vi "TiePie.Scp.ScpIsRunning.vi"(8 "error in (no error)":errorcluster, 11 "GenHandle":T1) -> (0 "error out":errorcluster, 2 "return type":u8, 3 "GenHandle out":T1)   [LabVIEW 2014, in "LVTiePie.lvlib"]
uses:
  LVTiePie.lvlib
  TiePie.Gen.handle.ctl
  bin/libtiepie.dll
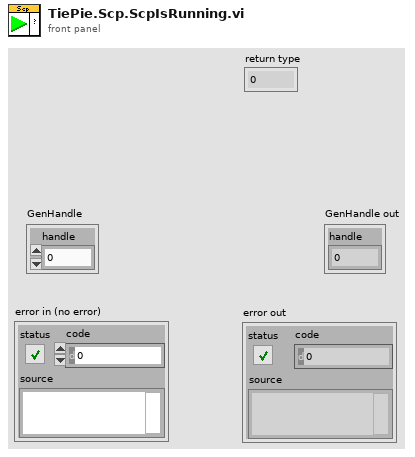
[diagram p1: front panel]
types:
  T1 = typedef "TiePie.Gen.handle.ctl" = cluster{"handle":u32}
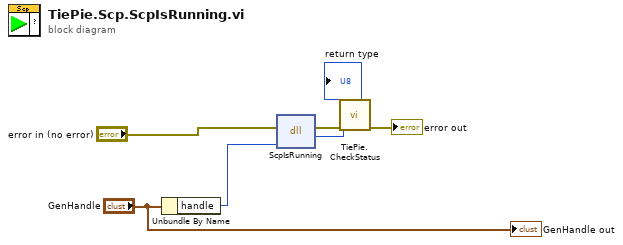
[diagram p0: block diagram]
diagram:
  n1 = Unbundle By Name("GenHandle") -> ("handle"=w5:u32)
  n2 = dll-call lib="C:/Users/mbirski/Desktop/PAN/LabVEW/Tie Pie/bin/libtiepie.dll" fn="ScpIsRunning"(error in="error in (no error)", "handle"=w5) -> (error out=w3:errorcluster, "return type"=→"return type":u8)  [unwired: 3 in, 1 out]
  n3 = call "TiePie.CheckStatus.vi"("error in (no error)"=w3) -> ("error out"=→"error out":errorcluster)  [unwired: 10 in]
  "GenHandle out" <- "GenHandle"
